vi "Rtn Rx Cal Para.vi"(6 "chain":u32, 7 "inputSignalStrength_dBm":i32, 8 "error in (no error)":errorcluster, 9 "numPackets":u32, 10 "rate":u32, 11 "freq":u32) -> (0 "error out":errorcluster, 3 "Rx Cal Parameter":T1)   [LabVIEW 2013, in "QCAWLAN_DLL.lvlib"]
uses:
  QCAWLAN_DLL.lvlib
  QCAWLAN_DLL.dll
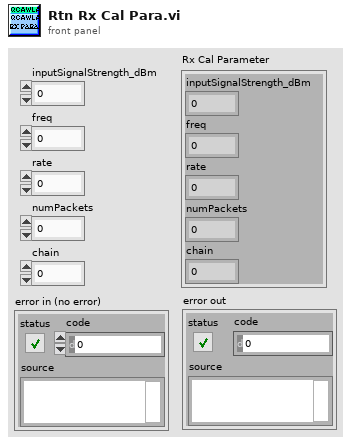
[diagram p1: front panel]
types:
  T1 = cluster{"inputSignalStrength_dBm":i32, "freq":u32, "rate":u32, "numPackets":u32, "chain":u32}
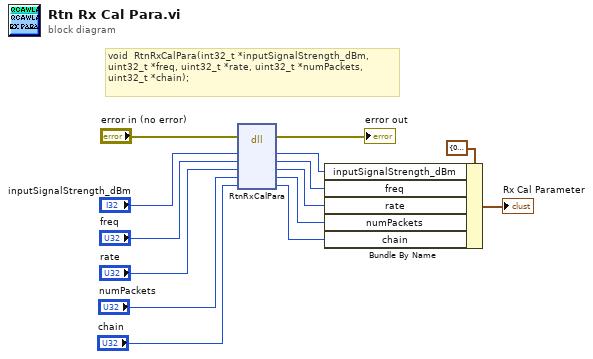
[diagram p0: block diagram]
diagram:
  # "void  RtnRxCalPara(int32_t *inputSignalStrength_dBm, uint32_t *freq, uint32_t *rate, uint32_t *numPackets, uint32_t *chain);"
  n1 = dll-call lib="C:/Connectivity Client - MIMO/PlugIn/QCAWLAN_DLL.dll" fn="RtnRxCalPara"(error in="error in (no error)", "inputSignalStrength_dBm"="inputSignalStrength_dBm", "freq"="freq", "rate"="rate", "numPackets"="numPackets", "chain"="chain") -> (error out=→"error out":errorcluster, "inputSignalStrength_dBm"=w9:i32, "freq"=w7:u32, "rate"=w6:u32, "numPackets"=w5:u32, "chain"=w4:u32)  [unwired: 3 in, 1 out]
  n2 = Bundle By Name(cluster=T1 {"inputSignalStrength_dBm"=0, "freq"=0, "rate"=0, "numPackets"=0, "chain"=0} ("Cluster 2"), "inputSignalStrength_dBm"=w9, "freq"=w7, "rate"=w6, "numPackets"=w5, "chain"=w4) -> (→"Rx Cal Parameter":T1)
